vi "biphasic_pulse.vi"() -> ()   [LabVIEW 2013]
panel:
  out "Waveform Graph":dbl[](graph)
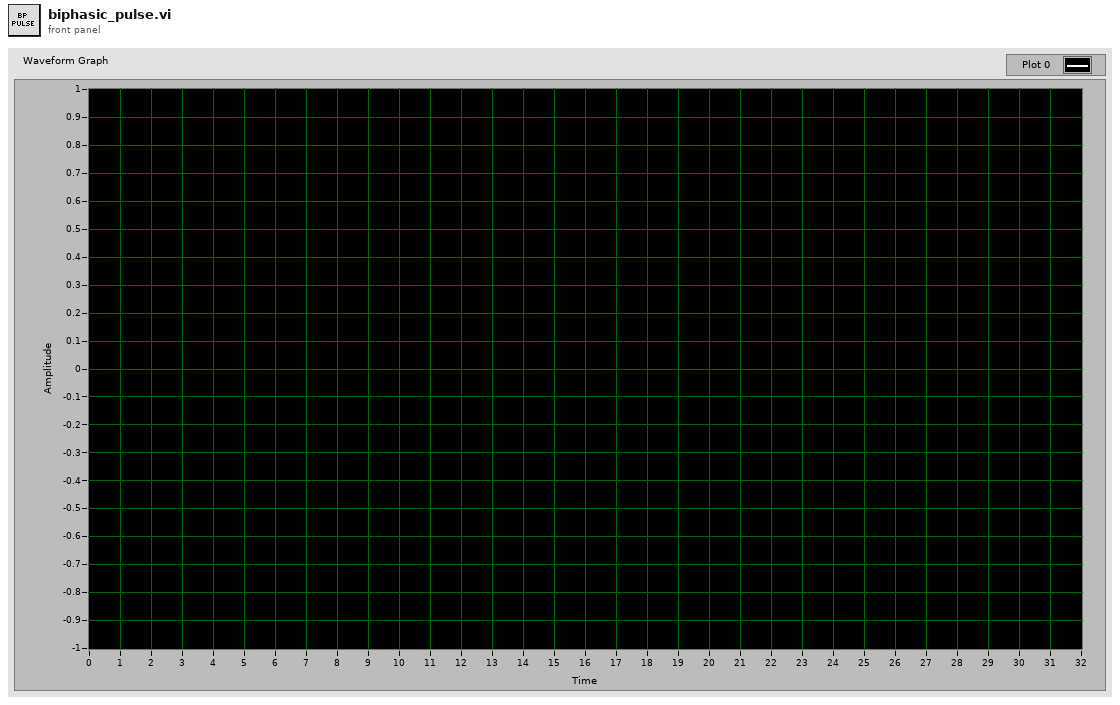
[diagram p1: front panel]
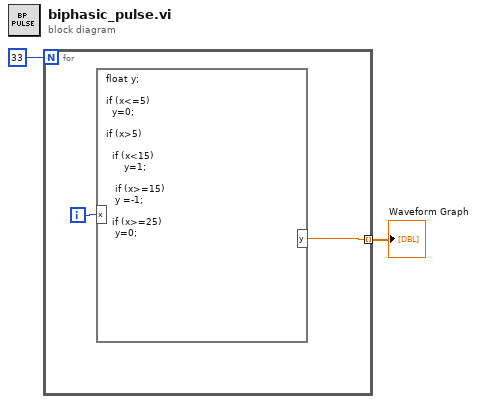
[diagram p0: block diagram]
diagram:
  n1 = for {
    N: 33 -> [_]
    tunnel: [w3] -> w1 mode=indexing
    i -> [w4]
    n2 = formula code="float y;\n\nif (x<=5)\n  y=0;\n\nif (x>5)\n\n  if (x<15)\n      y=1;\n\n   if (x>=15)\n   y =-1;\n\n  if (x>=25)\n   y=0;"("x"=w4) -> ("y"=w3:dbl)
  }
  "Waveform Graph" <- w1
